vi "Test_Average_Reactor_Cool_Loop_ACT_actual_derivative.vi"() -> ()   [LabVIEW 2022 SP3]
uses:
  SI_modules/SI101/SI101.lvclass
panel:
  out "Outputs":cluster{"Time":timestamp[], dbl[]}[](graph)
  out "Inputs":cluster{"Time":timestamp[], dbl[]}[](graph)
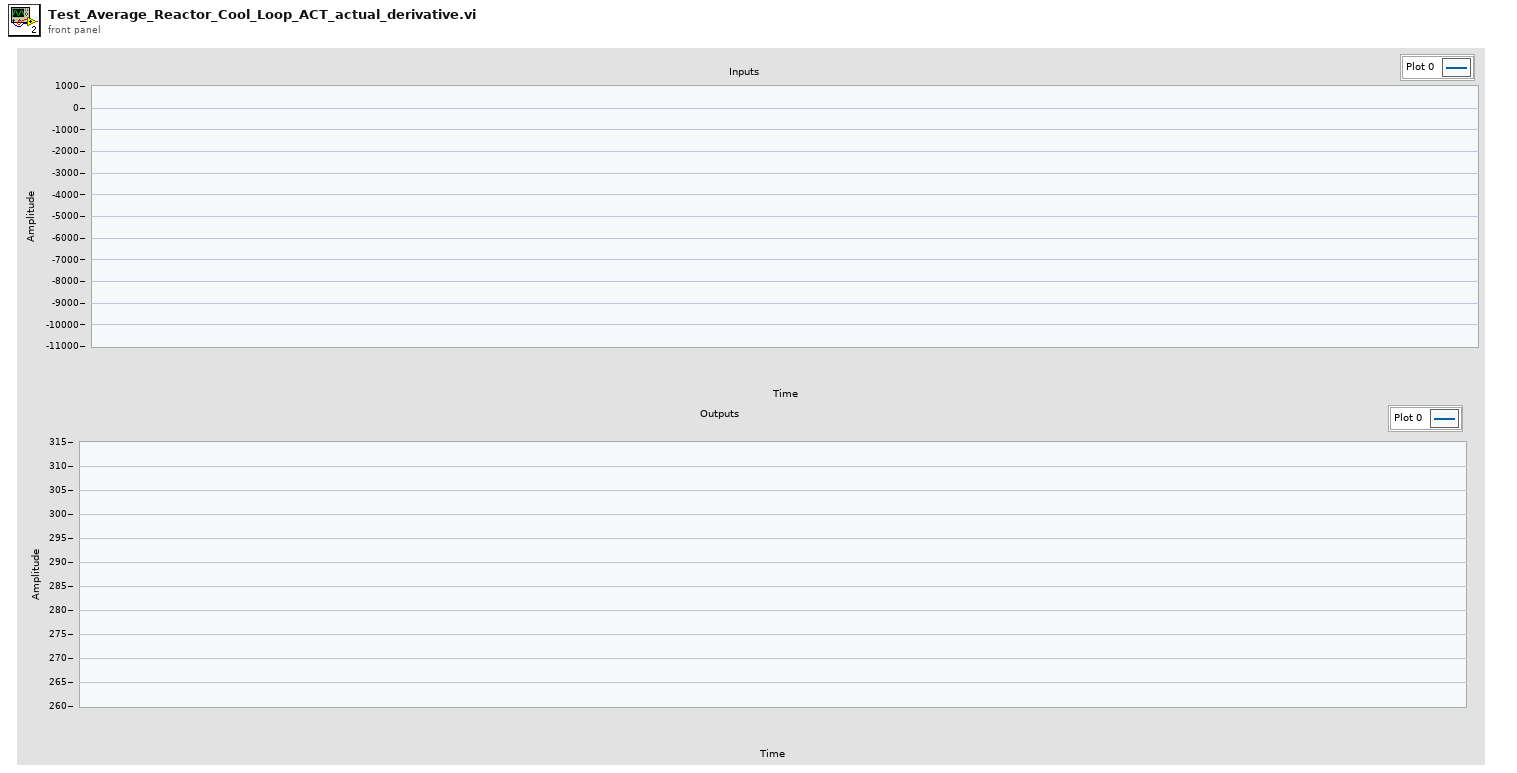
[diagram p1: front panel]
types:
  T1 = cluster{"[0]":cluster{"Time":timestamp[], "KKS":string, "Meas":dbl[]}, "[1]":cluster{"Time":timestamp[], "KKS":string, "Meas":dbl[]}, "[2]":cluster{"Time":timestamp[], "KKS":string, "Meas":dbl[]}, "[3]":cluster{"Time":timestamp[], "KKS":string, "Meas":dbl[]}, "[4]":cluster{"Time":timestamp[], "KKS":string, "Meas":dbl[]}, "[5]":cluster{"Time":timestamp[], "KKS":string, "Meas":dbl[]}, "[6]":cluster{"Time":timestamp[], "KKS":string, "Meas":dbl[]}, "[7]":cluster{"Time":timestamp[], "KKS":string, "Meas":dbl[]}, "[8]":cluster{"Time":timestamp[], "KKS":string, "Meas":dbl[]}}
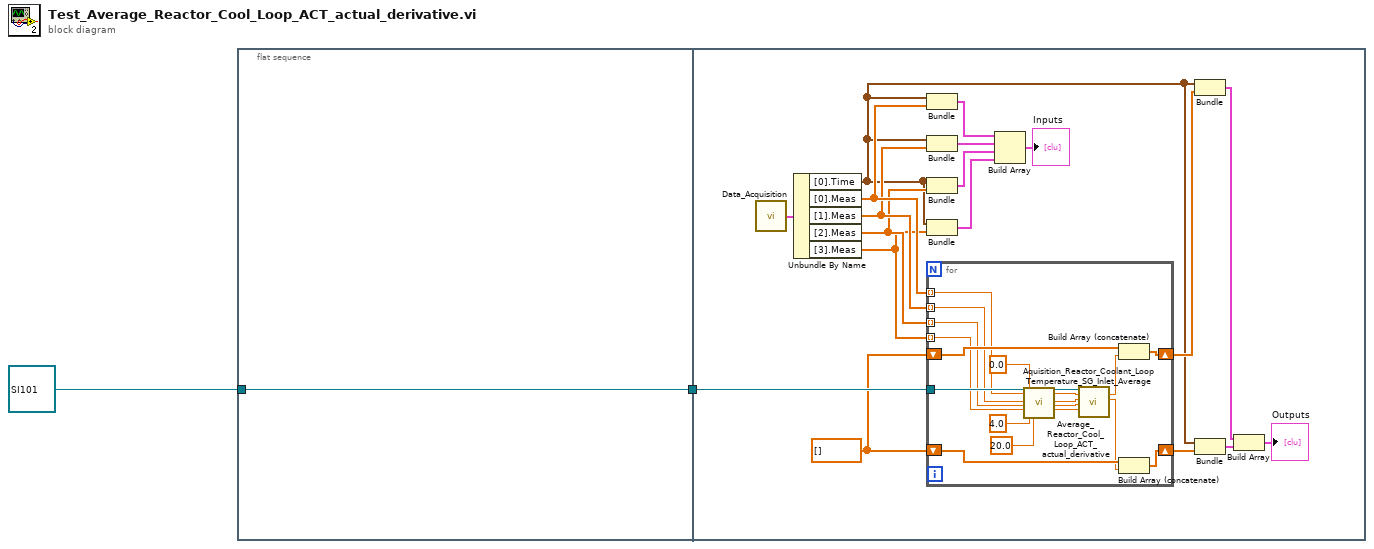
[diagram p0: block diagram]
diagram:
  n1 = flat-sequence {
    tunnel: refnum<class "SI101.lvclass"> refnum ("SI101_AverageReactorCoolantTemperature.lvclass") -> [w3]
    tunnel: [w3] -> w1
    tunnel: w1 -> [w10]
    frame #0 {
    }
    frame #1 {
      w9 = dbl[] []
      n2 = call "Data_Acquisition.vi"() -> ("Meas"=w21:T1)  [unwired: 15 in]
      n3 = Unbundle By Name(w21) -> ("[0].Time"=w7:timestamp[], "[0].Meas"=w20:dbl[], "[1].Meas"=w19:dbl[], "[2].Meas"=w18:dbl[], "[3].Meas"=w17:dbl[])
      n4 = Bundle("Time"=w7, "Meas"=w20) -> (w16:cluster{"Time":timestamp[], "Meas":dbl[]})  [unwired: 1 in]
      n5 = Bundle("Time"=w7, "Meas"=w19) -> (w15:cluster{"Time":timestamp[], "Meas":dbl[]})  [unwired: 1 in]
      n6 = Bundle("Time"=w7, "Meas"=w18) -> (w14:cluster{"Time":timestamp[], "Meas":dbl[]})  [unwired: 1 in]
      n7 = Bundle("Time"=w7, "Meas"=w17) -> (w13:cluster{"Time":timestamp[], "Meas":dbl[]})  [unwired: 1 in]
      n8 = for {
        tunnel: w20 -> [w38] mode=indexing
        tunnel: w19 -> [w37] mode=indexing
        tunnel: w18 -> [w36] mode=indexing
        tunnel: w17 -> [w35] mode=indexing
        shift-right: [w30] -> w11
        shift-left: w9 -> [w40]
        tunnel: w10 -> [w39]
        shift-right: [w31] -> w8
        shift-left: w9 -> [w32]
        n9 = call "Aquisition_Reactor_Coolant_Loop Temperature_SG_Inlet_Average.vi"("SI101_AverageReactorCoolantTemperature.lvclass"=w39, "3 JEC10 CT001B XQ01"=w38, "3 JEC20 CT001B XQ01"=w37, "3 JEC30 CT001B XQ01"=w36, "3 JEC40 CT001B XQ01"=w35, "SI100 Avg Temp Rise"=0.0, "In1"=4.0, "In2"=20.0) -> ("SI101_AverageReactorCoolantTemperature.lvclass out"=w28:refnum<class "SI101.lvclass">, "ACT Loop 1"=w27:dbl, "ACT Loop 2"=w26:dbl, "ACT loop 3"=w25:dbl, "ACT loop 4"=w24:dbl)  [unwired: 14 in, 1 out]
        n10 = call "Average_Reactor_Cool_Loop_ACT_actual_derivative.vi"("SI101_AverageReactorCoolantTemperature.lvclass"=w28, "ACT Loop1"=w27, "ACT Loop2"=w26, "ACT Loop3"=w25, "ACT Loop4"=w24) -> ("ACT 2nd Ctrl"=w22:dbl, "ACT D-Comp"=w23:dbl)  [unwired: 11 in, 2 out]
        n11 = Build Array (concatenate)(w40, w22) -> (w30:dbl[])
        n12 = Build Array (concatenate)(w32, w23) -> (w31:dbl[])
      }
      n13 = Build Array(w16, w15, w14, w13) -> (→"Inputs":cluster{"Time":timestamp[], "Meas":dbl[]}[])
      n14 = Bundle("Time"=w7, w11) -> (w6:cluster{"Time":timestamp[], dbl[]})  [unwired: 1 in]
      n15 = Bundle("Time"=w7, w8) -> (w5:cluster{"Time":timestamp[], dbl[]})  [unwired: 1 in]
      n16 = Build Array(w6, w5) -> (→"Outputs":cluster{"Time":timestamp[], dbl[]}[])
    }
  }
